vi "Fetch Waveform.vi"(4 "Sparsing (0: Every point)":i32, 5 "Number of points (0: All points)":i32, 6 "Segment number (0: All segment)":i16, 7 "First point (0: First point)":i32, 8 "error in (no error)":errorcluster, 9 "Timeout (10000 ms)":u32=10000, 10 "Source (1: Channel 1)":u16(ring)=1 items=["Channel 1"=1, "Channel 2"=2, "Channel 3"=3, "Channel 4"=4], 11 "VISA resource name":refnum<visa-resource-name>) -> (0 "error out":errorcluster, 2 "Waveform Graph":waveform(dbl)(graph), 3 "VISA resource name out":refnum<visa-resource-name>)   [LabVIEW 2021, in "Siglent SDS 1000 2000 Series.lvlib"]
doc: "Returns the waveform the oscilloscope acquired for the specified channel. The waveform is from an acquisition that you initiate prior to calling this VI.\n\nYou use the Initiate VI to start an acquisition on the channels that you enable with the <B>Configure Channel</B> VI. The oscilloscope acquires waveforms for the enabled channels concurrently. You must call this VI separately for each enabled channel to obtain the waveforms.\n\nYou can call the <B> Read Single Waveform</B> VI or <B> Read Multiple Waveforms</B> VI instead of using low level VIs.\n\n<B>Note</B> This VI does not check the instrument status. Typically, you call this VI only in a sequence of calls to other low-level instrument driver VIs. The sequence performs one operation. You use the low-level VIs to optimize one or more aspects of interaction with the instrument."
uses:
  <instrlib>/Siglent SDS 1000 2000 Series/Siglent SDS 1000 2000 Series.lvlib
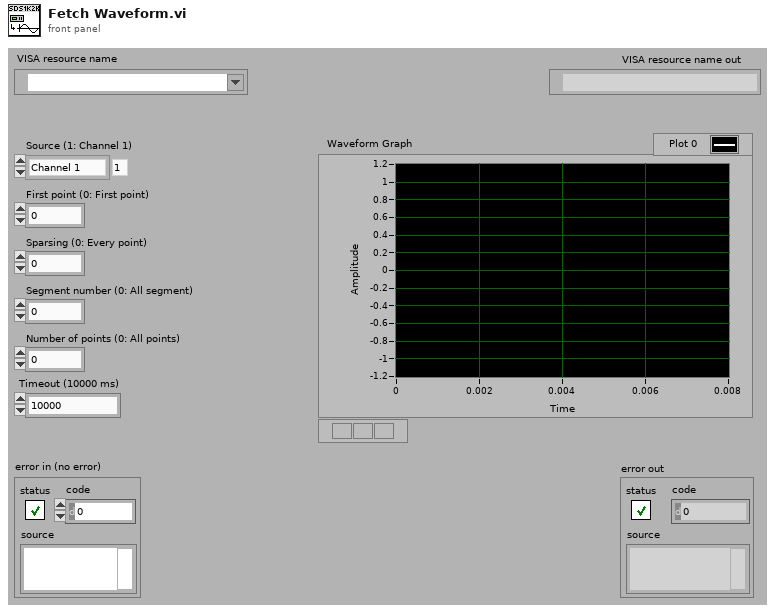
[diagram p1: front panel]
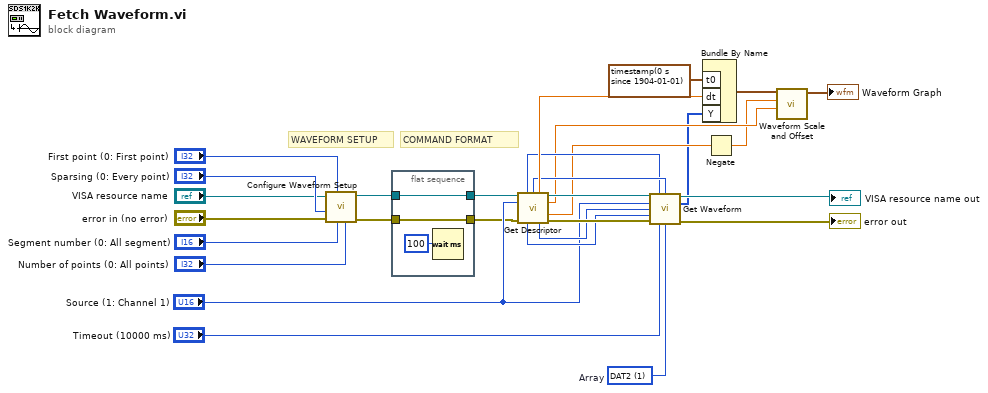
[diagram p0: block diagram]
diagram:
  w20 = u16 1 items=["DAT1", "DAT2"]  # Array
  # "WAVEFORM SETUP"
  # "COMMAND FORMAT"
  n1 = call <instrlib>:"Configure Waveform Setup.vi"("Number of points (0: All points)"="Number of points (0: All points)", "Segment number (0: All segment)"="Segment number (0: All segment)", "First point (0: First point)"="First point (0: First point)", "error in (no error)"="error in (no error)", "Sparsing (0: Every point)"="Sparsing (0: Every point)", "VISA resource name"="VISA resource name") -> ("error out"=w2:errorcluster, "VISA resource name out"=w4:refnum<visa-resource-name>)  [unwired: 4 in]
  n2 = flat-sequence {
    tunnel: w4 -> [w32]
    tunnel: [w32] -> w3
    tunnel: w2 -> [w31]
    tunnel: [w31] -> w1
    frame #0 {
      n3 = Wait (ms)(milliseconds to wait=100) -> ()  [unwired: 1 out]
    }
  }
  n4 = call <instrlib>:"Get Descriptor.vi"("VISA resource name"=w3, "Source (1: Channel 1)"="Source (1: Channel 1)", "error in (no error)"=w1) -> ("First Valid Point"=w16:i32, "Last Valid Point"=w17:i32, "Horizontal interval"=w21:sgl, "VISA resource name out"=w29:refnum<visa-resource-name>, "Vertical gain"=w13:sgl, "Vertical offset"=w12:sgl, "Number Of Data Points"=w19:i32, "Command type"=w25:i16, "error out"=w28:errorcluster)  [unwired: 2 in, 2 out]
  n5 = call <instrlib>:"Get Waveform.vi"("VISA resource name"=w29, "First Valid Point"=w16, "Last Valid Point"=w17, "Source (1: Channel 1)"="Source (1: Channel 1)", "Command type (0: byte)"=w25, "Number Of Data Points (10000)"=w19, "error in (no error)"=w28, "Timeout (10000 ms)"="Timeout (10000 ms)", "Array (0: DAT1)"=w20) -> ("VISA resource name out"=→"VISA resource name out":refnum<visa-resource-name>, "Waveform Graph"=w6:i16[], "error out"=→"error out":errorcluster)  [unwired: 4 in]
  n6 = Bundle By Name ("Build Waveform")("t0"=timestamp(0 s since 1904-01-01), "dt"=w21, "Y"=w6) -> (w15:waveform(i16))  [unwired: 1 in]
  n7 = Negate(x=w12) -> (-x=w11:sgl)
  n8 = call <vilib>:"Waveform Scale and Offset.vi"("scale"=w13, "offset"=w11, "waveform in"=w15) -> ("waveform out"=→"Waveform Graph":waveform(dbl))  [unwired: 7 in, 1 out]
